vi "Write Rescale Configuration.vi"(8 "error in (no error)":errorcluster, 10 "Configuration":T1, 11 "Rescale in":refnum<class "Rescale.lvclass">) -> (0 "error out":errorcluster, 3 "Rescale out":refnum<class "Rescale.lvclass">)   [LabVIEW 2018, in "Rescale.lvclass"]
uses:
  Rescale.lvclass
  C:/github/LabActor/Template Module/Template Module.lvclass
  Rescale Configuration.ctl
  NHMFL_Core/Libraries/File/Controls/NXG TDMS channel re-scale selector entry.ctl
  Template Module/Template Module.lvclass/Template Module.ctl
  Template Module/Write Configuration.vi
panel:
  # "Use   Group                     Channel                               New channel                                Scale"
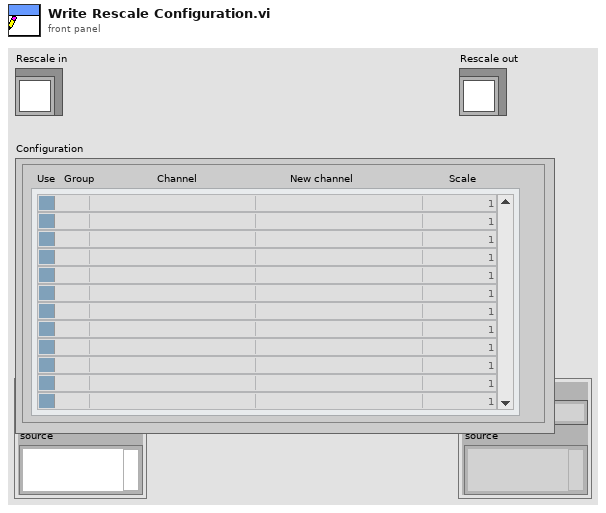
[diagram p1: front panel]
types:
  T1 = typedef "Rescale Configuration.ctl" = cluster{"Channels":T2[]}
  T2 = typedef "NXG TDMS channel re-scale selector entry.ctl" = cluster{"Group":string, "Channel":string, "Active":bool, "New channel":string, "Re-scale factor":dbl}
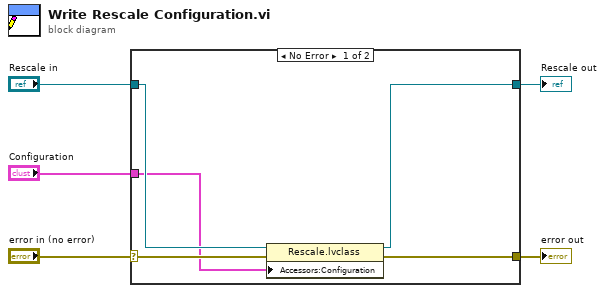
[diagram p0: block diagram]
diagram:
  n1 = case shown="No Error" "error in (no error)" {
    selector: "error in (no error)" -> [w10 w11]
    tunnel: [w9 w11] -> w4
    tunnel: [w7 w12] -> w2
    tunnel: "Rescale in" -> [w8 w12]
    tunnel: "Configuration" -> [w6 _]
    frame No Error {
      n2 = property class="Rescale.lvclass"(reference=w8, error in=w10, "Accessors:Configuration"=w6) -> (reference out=w7:refnum<class "Rescale.lvclass">, error out=w9:errorcluster)
    }
    frame Error {
    }
  }
  "error out" <- w4
  "Rescale out" <- w2
